vi "Unit Test empty BlueSerializable.vi"() -> ()   [LabVIEW 2019, in "Sports Unit Tests.lvclass"]
uses:
  Sports Unit Tests.lvclass
  <userlib>/Blue Origin/BlueSerialization/BlueSerializable/BlueSerializable.lvclass
  <vilib>/Utility/error.llb/Clear Errors.vi
  <vilib>/addons/_JKI Toolkits/Caraya/classes/Test/Define Test.vi
  <vilib>/addons/_JKI Toolkits/Caraya/classes/Assert/Assert Equal Value_Variant.vi
  <vilib>/addons/_JKI Toolkits/Caraya/classes/Assert/Assert Not Error.vi
  <vilib>/addons/_JKI Toolkits/Caraya/classes/Assert/Assert.lvclass
  <userlib>/Blue Origin/BlueSerialization/BlueSerializer/BlueSerializer.lvclass
panel:
  out "Table":string[][](table)
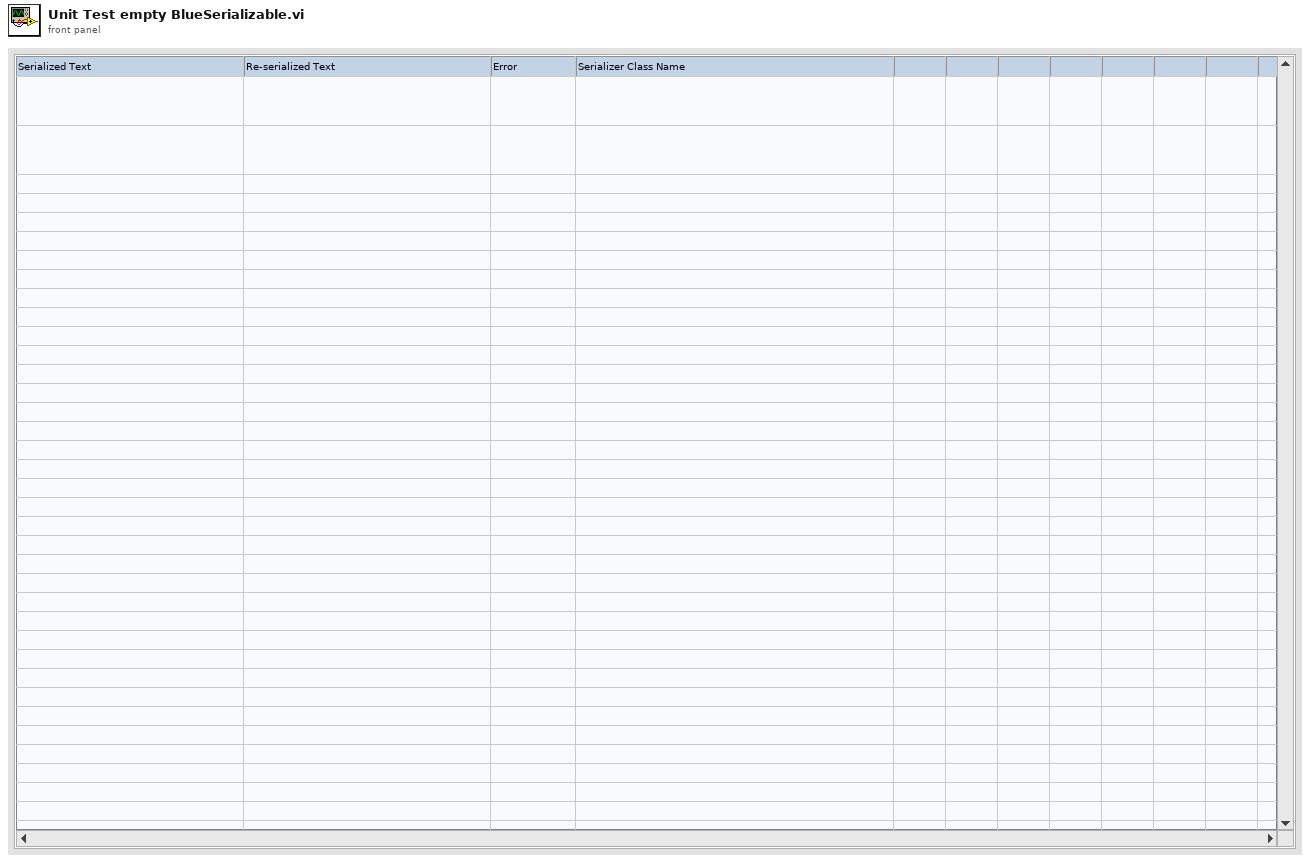
[diagram p1: front panel]
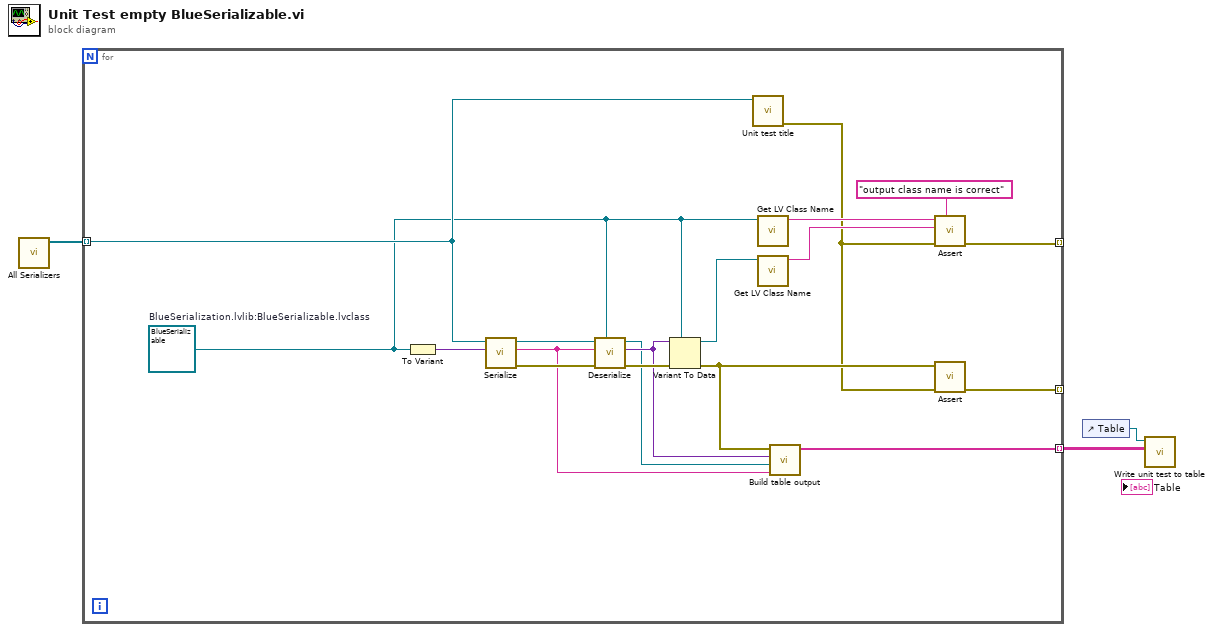
[diagram p0: block diagram]
diagram:
  n1 = call "All Serializers.vi"() -> ("All serializers"=w2:refnum<class "BlueSerializer.lvclass">[])  [unwired: 11 in]
  n2 = for {
    tunnel: w2 -> [w8] mode=indexing
    tunnel: [w13] -> _ mode=indexing
    tunnel: [w9] -> w1 mode=indexing
    tunnel: [w5] -> _ mode=indexing
    w4 = refnum<class "BlueSerializable.lvclass"> refnum  # BlueSerialization.lvlib:BlueSerializable.lvclass
    n3 = To Variant(anything=w4) -> (Variant=w19:variant)
    n4 = call <userlib>:"Serialize.vi"("Anything"=w19, "BlueSerializer in"=w8) -> ("error out"=w21:errorcluster, "Serialized Text"=w10:string, "BlueSerializer out"=w20:refnum<class "BlueSerializer.lvclass">)  [unwired: 7 in]
    n5 = call <userlib>:"Deserialize.vi"("Anything"=w4, "error in (no error)"=w21, "Serialized Text"=w10, "BlueSerializer in"=w20) -> ("error out"=w18:errorcluster, "Variant"=w12:variant, "BlueSerializer out"=w11:refnum<class "BlueSerializer.lvclass">)  [unwired: 5 in]
    n6 = Variant To Data(error in=w18, type=w4, Variant=w12) -> (data=w17:refnum<class "BlueSerializable.lvclass">, error out=w7:errorcluster)
    n7 = call "Unit test title.vi"("serializer"=w8) -> ("error out"=w6:errorcluster)  [unwired: 9 in, 1 out]
    n8 = call <vilib>:"Get LV Class Name.vi"("object"=w4) -> ("class name"=w16:string)  [unwired: 9 in, 1 out]
    n9 = call <vilib>:"Get LV Class Name.vi"("object"=w17) -> ("class name"=w15:string)  [unwired: 9 in, 1 out]
    n10 = call "Build table output.vi"("serialized text"=w10, "BlueSerializer in"=w11, "deserialized variant"=w12, "variant to data error"=w7) -> ("table output"=w9:string[])  [unwired: 7 in]
    n11 = call-poly <vilib>:"Assert.vi"("Label"="output class name is correct", "error in (no error)"=w6, "Y"=w15, "X"=w16) -> ("error out"=w13:errorcluster)  [unwired: 7 in]
    n12 = call-poly <vilib>:"Assert.vi"("error in (no error)"=w6, "Not Error?"=w7) -> ("error out"=w5:errorcluster)  [unwired: 9 in]
  }
  n13 = control-ref of="Table"() -> (w3:refnum<vi>)
  n14 = call "Write unit test to table.vi"("Table"=w1, "Table ref in"=w3) -> ()  [unwired: 9 in, 1 out]
